vi "C4LV_openDevice.vi"(0 "c4if Arr in":refnum<k24>[](array[refnum]), 5 "devName in":string, 11 "error in (no error)":errorcluster) -> (4 "c4if Arr out":refnum<k24>[](array[refnum]), 6 "c4dev out":refnum<k24>, 15 "error out":errorcluster)   [LabVIEW 2015, in "libC4HdlLV.lvlib"]
uses:
  libC4HdlLV.lvlib
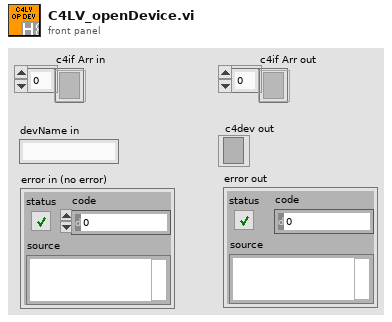
[diagram p1: front panel]
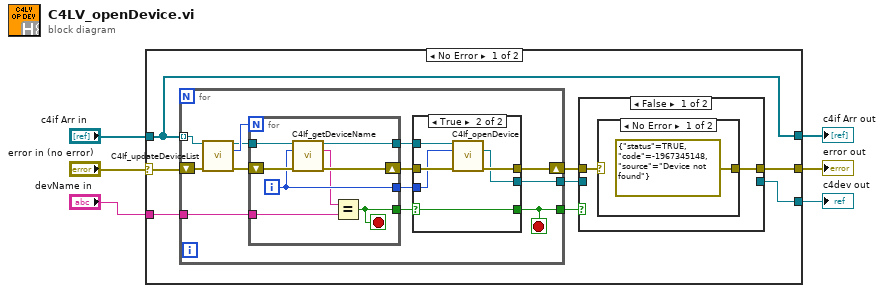
[diagram p0: block diagram]
diagram:
  n1 = case shown="No Error" "error in (no error)" {
    selector: "error in (no error)" -> [w8 w51]
    tunnel: "devName in" -> [w14 _]
    tunnel: [w13 w51] -> w5
    tunnel: [w9 _] -> w1
    tunnel: "c4if Arr in" -> [w7 w50]
    tunnel: [w7 w50] -> w2
    frame No Error {
      n2 = for {
        tunnel: w7 -> [w22] mode=indexing
        tunnel: w14 -> [w29]
        tunnel: [w28] -> w10
        tunnel: [w27] -> w12
        shift-right: [w26] -> w11
        shift-left: w8 -> [w25]
        stop <- w27 stop-if-true
        n3 = call "C4If_updateDeviceList.vi"("c4if in"=w22, "error in (no error)"=w25) -> ("c4if out"=w21:refnum<k24>, "nofDev out"=w23:i64, "error out"=w24:errorcluster)  [unwired: 11 in]
        n4 = for {
          N: w23 -> [_]
          tunnel: w21 -> [w45]
          shift-right: [w46] -> w33
          shift-left: w24 -> [w47]
          tunnel: [w49] -> w30
          tunnel: [w43] -> w32
          tunnel: [w44] -> w31
          tunnel: w29 -> [w48]
          i -> [w44]
          stop <- w49 stop-if-true
          n5 = call "C4If_getDeviceName.vi"("c4if in"=w45, "devNo in"=w44, "error in (no error)"=w47) -> ("c4if out"=w43:refnum<k24>, "device name out"=w42:string, "error out"=w46:errorcluster)  [unwired: 10 in]
          n6 = Equal?(x=w42, y=w48) -> (x = y?=w49:bool)
        }
        n7 = case shown="True" w30 {
          selector: w30 -> [w35 w41]
          tunnel: w33 -> [w34 w39]
          tunnel: w32 -> [_ w40]
          tunnel: w31 -> [_ w38]
          tunnel: [_ w36] -> w28
          tunnel: [w35 w41] -> w27
          tunnel: [w34 w37] -> w26
          frame False {
          }
          frame True {
            n8 = call "C4If_openDevice.vi"("c4if in"=w40, "devNo in"=w38, "error in (no error)"=w39) -> ("c4dev out"=w36:refnum<k24>, "error out"=w37:errorcluster)  [unwired: 10 in, 1 out]
          }
        }
      }
      n9 = case shown="False" w12 {
        tunnel: w11 -> [w16 w20]
        tunnel: [w15 w20] -> w13
        tunnel: w10 -> [_ w19]
        tunnel: [_ w19] -> w9
        frame False {
          n10 = case shown="No Error" w16 {
            selector: w16 -> [_ w18]
            tunnel: [errorcluster {"status"=TRUE, "code"=-1967345148, "source"="Device not found"} ("error out") w18] -> w15
            frame No Error {
            }
            frame Error {
            }
          }
        }
        frame True {
        }
      }
    }
    frame Error {
    }
  }
  "error out" <- w5
  "c4if Arr out" <- w2
  "c4dev out" <- w1
